vi "MatchProject&GiveLogFile-FileName&Format.vi"(11 "ProjectIndex":i32) -> (2 "CUST P/N":string, 3 "FCT_LOG":string)   [LabVIEW 2018]
panel:
  out "String":string
  in  "Cleaned Array":string[](array[string])
  out "Array":string[](array[string])
  out "FileName&Format-NoHeader":string
  out "FileName&Format":string
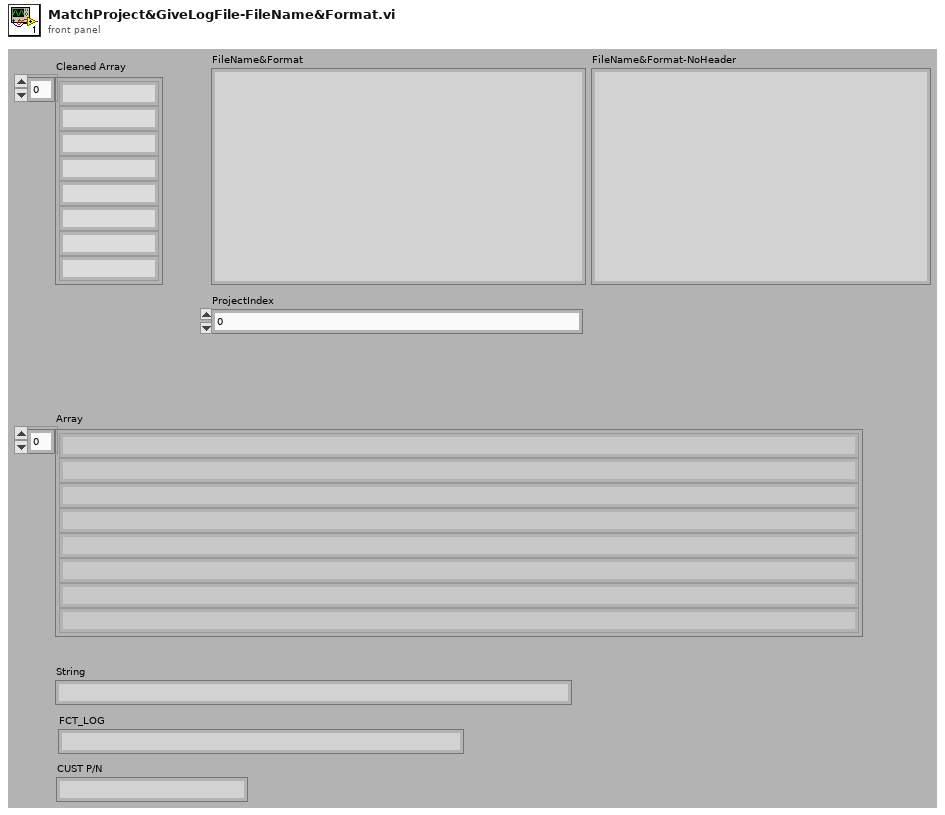
[diagram p1: front panel]
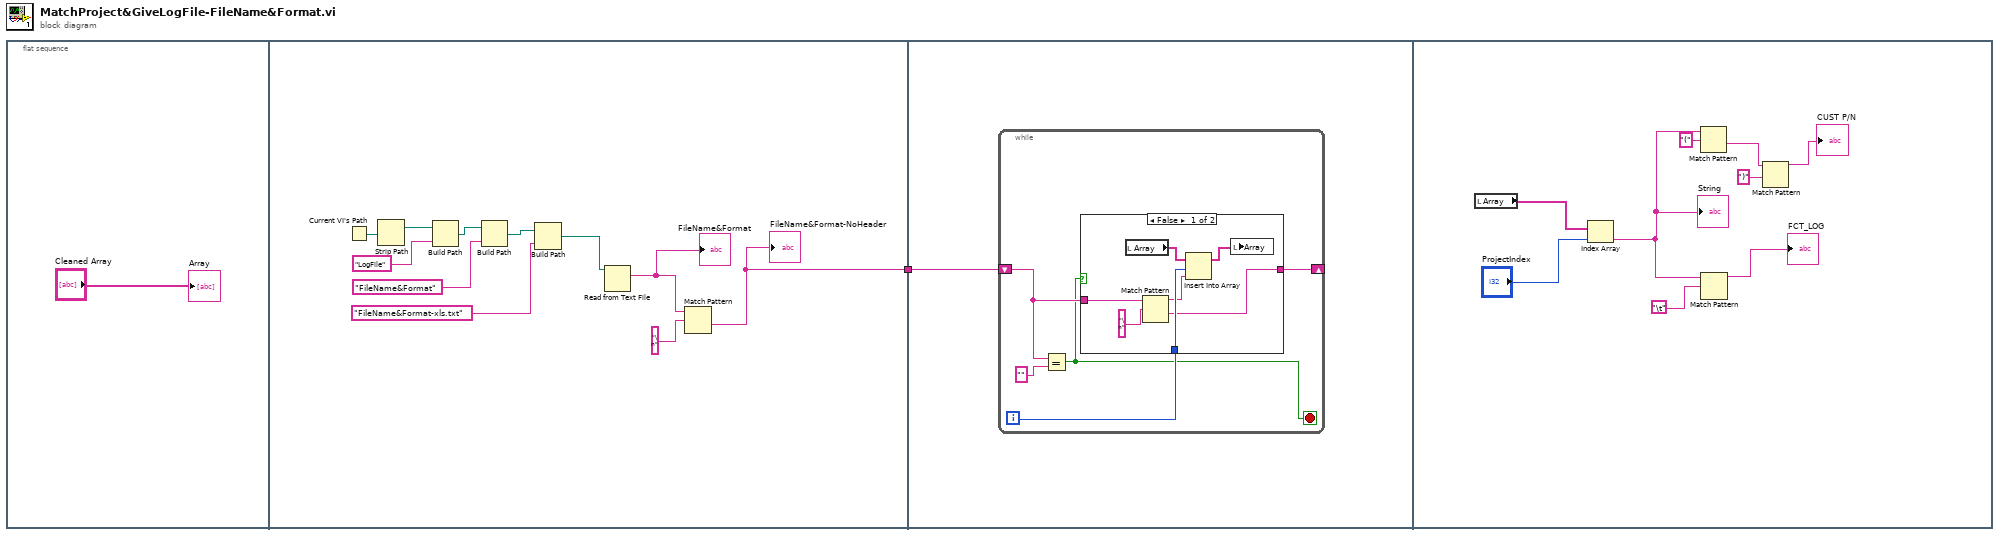
[diagram p0: block diagram]
diagram:
  n1 = flat-sequence {
    tunnel: [w3] -> w1
    tunnel: w1 -> [w14]
    frame #0 {
      "Array" <- "Cleaned Array"
    }
    frame #1 {
      n2 = Current VI's Path() -> (path=w9:path)
      n3 = Strip Path(path=w9) -> (stripped path=w10:path)  [unwired: 1 out]
      n4 = Build Path(base path=w10, name or relative path="LogFile") -> (appended path=w7:path)
      n5 = Build Path(base path=w7, name or relative path="FileName&Format") -> (appended path=w13:path)
      n6 = Build Path(base path=w13, name or relative path="FileName&Format-xls.txt") -> (appended path=w6:path)
      n7 = Read from Text File(file (use dialog)=w6) -> (text=w5:string)  [unwired: 1 in, 5 out]
      "FileName&Format" <- w5
      n8 = Match Pattern(string=w5, regular expression="\n") -> (after substring=w3:string)  [unwired: 4 out]
      "FileName&Format-NoHeader" <- w3
    }
    frame #2 {
      n9 = while {
        shift-right: [w18] -> _
        shift-left: w14 -> [w17]
        i -> [w19]
        stop <- w15 stop-if-true
        n10 = Equal?(x=w17, y="" ("regular expression")) -> (x = y?=w15:bool)
        n11 = case shown="False" w15 {
          tunnel: w19 -> [w24 _]
          tunnel: [w22 w27] -> w18
          tunnel: w17 -> [w21 w27]
          frame False {
            n12 = local read "Array"() -> (w20:string[])
            n13 = Match Pattern(string=w21, regular expression="\n") -> (before substring=w23:string, after substring=w22:string)  [unwired: 3 out]
            n14 = Insert Into Array(array=w20, index=w24, new element=w23) -> (w25:string[])
            n15 = local write "Array"(w25) -> ()
          }
          frame True {
          }
        }
      }
    }
    frame #3 {
      n16 = local read "Array"() -> (w36:string[])
      n17 = Index Array(array=w36, index="ProjectIndex") -> (element=w32:string)
      "String" <- w32
      n18 = Match Pattern(string=w32, regular expression="(") -> (after substring=w30:string)  [unwired: 4 out]
      n19 = Match Pattern(string=w32, regular expression="\t") -> (before substring=→"FCT_LOG":string)  [unwired: 4 out]
      n20 = Match Pattern(string=w30, regular expression=")") -> (before substring=→"CUST P/N":string)  [unwired: 4 out]
    }
  }
